vi "Open Excel File.vi"(8 "error in (no error)":errorcluster, 11 "File":path) -> (0 "error out":errorcluster, 3 "ExcelRefs":T1)   [LabVIEW 2011]
uses:
  Controls/Excel Refs.ctl
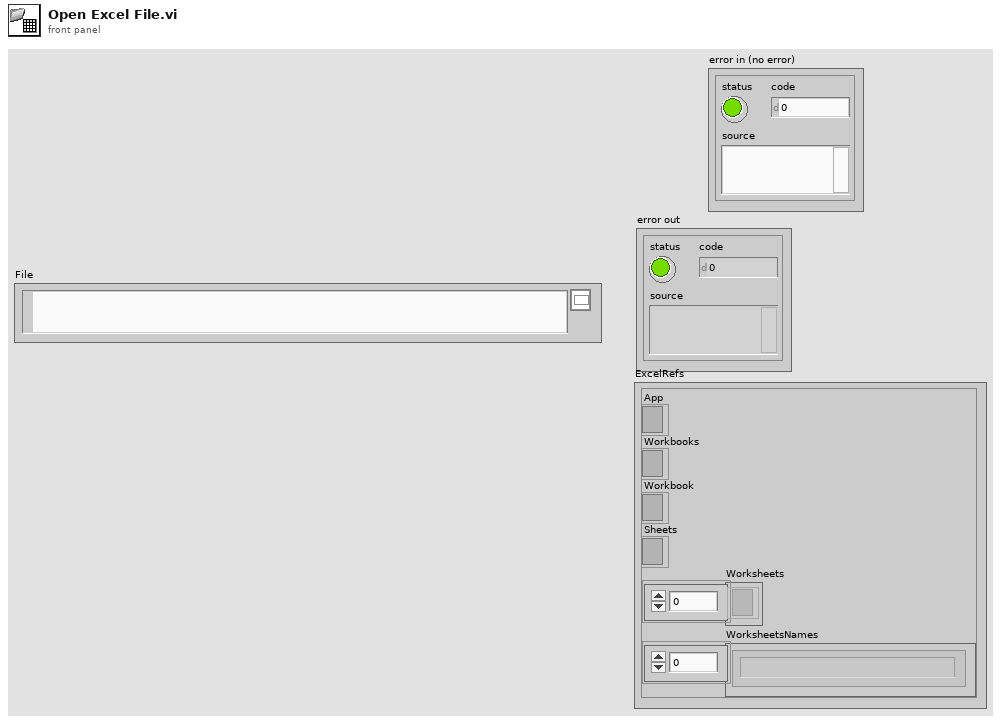
[diagram p1: front panel]
types:
  T1 = typedef "Excel Refs.ctl" = cluster{"App":refnum<k7>, "Workbooks":refnum<k7>, "Workbook":refnum<k7>, "Sheets":refnum<k7>, "Worksheets":refnum<k7>[], "WorksheetsNames":string[]}
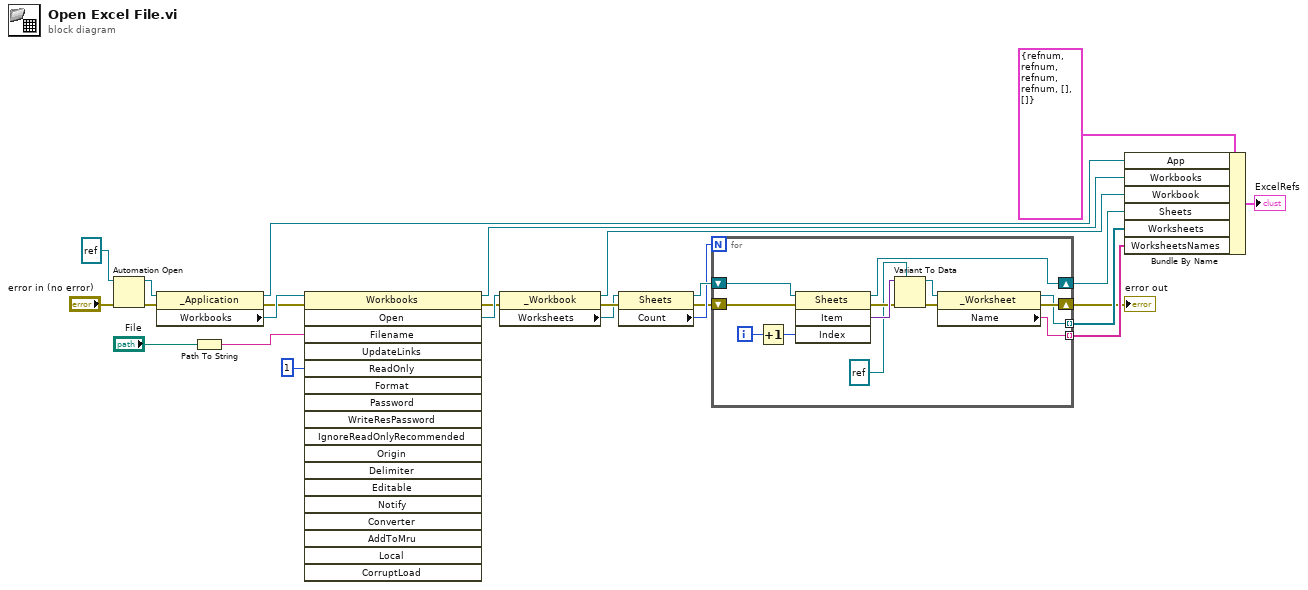
[diagram p0: block diagram]
diagram:
  n1 = Automation Open(error in (no error)="error in (no error)", Automation Refnum=refnum<k7> refnum ("Excel._Application")) -> (Automation Refnum=w15:refnum<k7>, error out=w25:errorcluster)  [unwired: 2 in]
  n2 = property class="_Application"(reference=w15, error in=w25) -> (reference out=w8:refnum<k7>, error out=w22:errorcluster, "Workbooks"=w23:refnum<k7>)
  n3 = Path To String(path="File") -> (string=w20:string)
  n4 = invoke class="Workbooks" method="Open"(reference=w23, error in=w22, "Filename"=w20, "ReadOnly"=1) -> (reference out=w7:refnum<k7>, error out=w17:errorcluster, "Open"=w18:refnum<k7>)  [unwired: 14 in, 15 out]
  n5 = property class="_Workbook"(reference=w18, error in=w17) -> (reference out=w6:refnum<k7>, error out=w16:errorcluster, "Worksheets"=w14:refnum<k7>)
  n6 = property class="Sheets"(reference=w14, error in=w16) -> (reference out=w13:refnum<k7>, error out=w11:errorcluster, "Count"=w12:i32)
  n7 = for {
    N: w12 -> [_]
    shift-right: [w37] -> w5
    shift-left: w13 -> [w38]
    shift-right: [w27] -> w2
    shift-left: w11 -> [w35]
    tunnel: [w29] -> w3 mode=indexing
    tunnel: [w26] -> w4 mode=indexing
    i -> [w36]
    n8 = Increment(x=w36) -> (x+1=w28:i32)
    n9 = invoke class="Sheets" method="Item"(reference=w38, error in=w35, "Index"=w28) -> (reference out=w37:refnum<k7>, error out=w33:errorcluster, "Item"=w34:variant)  [unwired: 1 in, 1 out]
    n10 = Variant To Data(error in=w33, type=refnum<k7> refnum ("Excel report.Excel._Worksheet"), Variant=w34) -> (data=w30:refnum<k7>, error out=w31:errorcluster)
    n11 = property class="_Worksheet"(reference=w30, error in=w31) -> (reference out=w26:refnum<k7>, error out=w27:errorcluster, "Name"=w29:string)
  }
  "error out" <- w2
  n12 = Bundle By Name(cluster=T1 {"App"=refnum, "Workbooks"=refnum, "Workbook"=refnum, "Sheets"=refnum, "Worksheets"=[], "WorksheetsNames"=[]} ("ExcelRefs"), "App"=w8, "Workbooks"=w7, "Workbook"=w6, "Sheets"=w5, "Worksheets"=w4, "WorksheetsNames"=w3) -> (→"ExcelRefs":T1)
